vi "calculate magnet voltage sequence.vi"(6 "Magnet Ramp Segments":string[][](array[string])) -> (0 "Magnet Voltage Sequence":dbl[](array[numeric]))   [LabVIEW 2014]
doc: "This VI accepts a table control containing rows of magnet ramp segments. Each segment consists of a start voltage, end voltage, and number of steps to take between those two voltages. The output in an interpolated array of voltages ready to be sent to the analogue input of a magnet power supply."
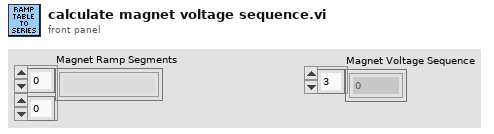
[diagram p1: front panel]
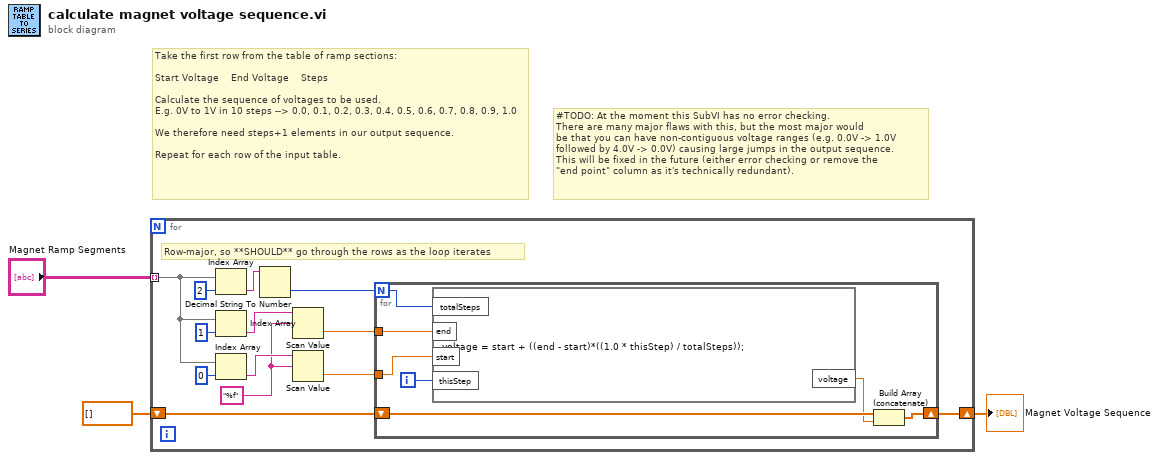
[diagram p0: block diagram]
diagram:
  # "#TODO: At the moment this SubVI has no error checking.\nThere are many major flaws with this, but the most major would\nbe that you can have non-contiguous voltage ranges (e.g. 0.0V -> 1.0V\nfollowed by 4.0V -> 0.0V) causing large jumps in the output sequence.\nThis will be fixed in the future (either error checking or remove the\n\"end point\" column as it's technically redundant)."
  # "Take the first row from the table of ramp sections:\n\nStart Voltage    End Voltage    Steps\n\nCalculate the sequence of voltages to be used.\nE.g. 0V to 1V in 10 steps --> 0.0, 0.1, 0.2, 0.3, 0.4, 0.5, 0.6, 0.7, 0.8, 0.9, 1.0\n\nWe therefore need steps+1 elements in our output sequence.\n\nRepeat for each row of the input table."
  n1 = for {
    tunnel: "Magnet Ramp Segments" -> [w12] mode=indexing
    shift-right: [w10] -> w1
    shift-left: dbl[] [] -> [w11]
    w5 = "%f" ("format string")
    # "Row-major, so **SHOULD** go through the rows as the loop iterates"
    n2 = Index Array(array=w12, index=2) -> (element=w13:string)
    n3 = Index Array(array=w12, index=1) -> (element=w4:string)
    n4 = Index Array(array=w12, index=0) -> (element=w8:string)
    n5 = Decimal String To Number(string=w13) -> (number=w9:i32)  [unwired: 2 in, 1 out]
    n6 = Scan Value(string=w4, format string=w5) -> (value=w6:dbl)  [unwired: 1 in, 1 out]
    n7 = Scan Value(string=w8, format string=w5) -> (value=w7:dbl)  [unwired: 1 in, 1 out]
    n8 = for {
      N: w9 -> [w23]
      tunnel: w6 -> [w22]
      tunnel: w7 -> [w21]
      shift-right: [w17] -> w10
      shift-left: w11 -> [w19]
      i -> [w20]
      n9 = formula code="voltage = start + ((end - start)*((1.0 * thisStep) / totalSteps));"("totalSteps"=w23, "end"=w22, "start"=w21, "thisStep"=w20) -> ("voltage"=w18:dbl)
      n10 = Build Array (concatenate)(w19, w18) -> (w17:dbl[])
    }
  }
  "Magnet Voltage Sequence" <- w1
